vi "read_attributes.vi"(8 "error in (no error)":errorcluster, 11 "LinearDiscriminantAnalysis in":refnum<class "LinearDiscriminantAnalysis.lvclass">) -> (0 "error out":errorcluster, 2 "attributes":T1, 3 "LinearDiscriminantAnalysis out":refnum<class "LinearDiscriminantAnalysis.lvclass">)   [LabVIEW 2020, in "LinearDiscriminantAnalysis.lvclass"]
uses:
  LinearDiscriminantAnalysis.lvclass
  Controls/linear_discriminant_analysis_attributes.ctl
  LinearDiscriminantAnalysis.lvclass/LinearDiscriminantAnalysis.ctl
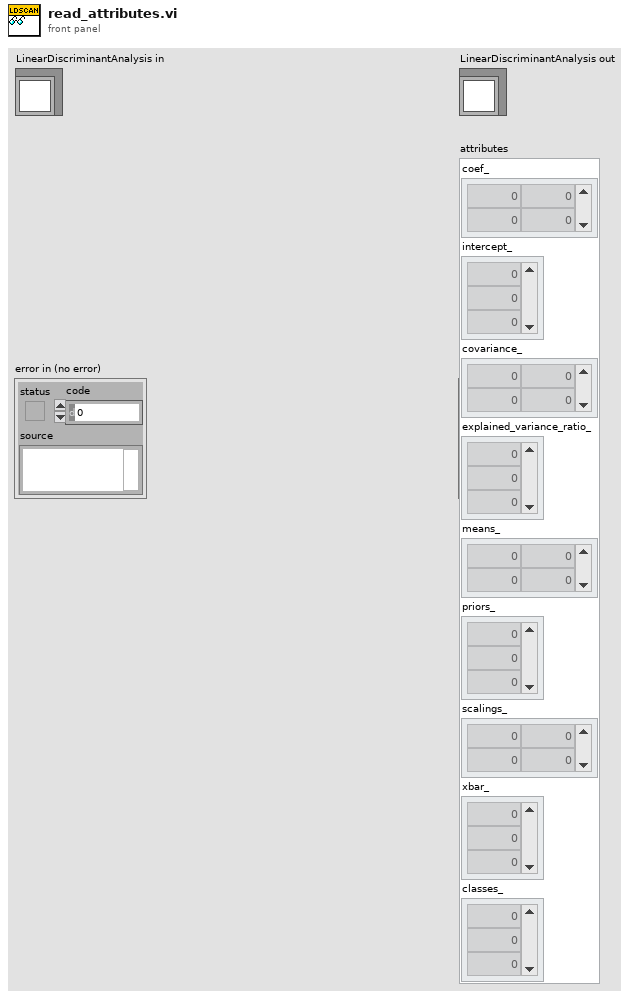
[diagram p1: front panel]
types:
  T1 = typedef "linear_discriminant_analysis_attributes.ctl" = cluster{"coef_":dbl[][], "intercept_":dbl[], "covariance_":dbl[][], "explained_variance_ratio_":dbl[], "means_":dbl[][], "priors_":dbl[], "scalings_":dbl[][], "xbar_":dbl[], "classes_":dbl[]}
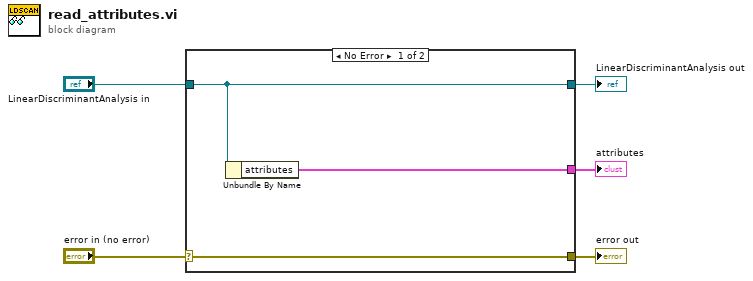
[diagram p0: block diagram]
diagram:
  n1 = case shown="No Error" "error in (no error)" {
    selector: "error in (no error)" -> [w8 w9]
    tunnel: [w8 w9] -> w4
    tunnel: [w7 w10] -> w2
    tunnel: "LinearDiscriminantAnalysis in" -> [w7 w10]
    tunnel: [w6 _] -> w1
    frame No Error {
      n2 = Unbundle By Name(w7) -> ("attributes"=w6:T1)
    }
    frame Error {
    }
  }
  "error out" <- w4
  "LinearDiscriminantAnalysis out" <- w2
  "attributes" <- w1
